vi "Assert To Report Entry.vi"(8 "error in (no error)":errorcluster, 10 "Assert Event Data":T1={"name"="", "passed"=FALSE, "call-chain"=[], "test-error"={"status"=FALSE, "code"=0, "source"=""}, "timestamp"=timestamp(0 s since 1904-01-01), "assert-id"="", "test-id"="", "time"=-1.0, "message"="", "properties"=variant, "measurements"=variant, "user-defined"=variant}) -> (0 "error out":errorcluster, 2 "String":string)   [LabVIEW 2020, in "Caraya.lvlib" / "Test Report.Event.lvclass"]
uses:
  Test Report.Event.lvclass
  Test Report.Event.lvclass/Test Report.Event.ctl
  Test Report/Test Report.lvclass
  Test Result/Assert Event Data (Extended).ctl
  Test Result/Test Result.lvclass
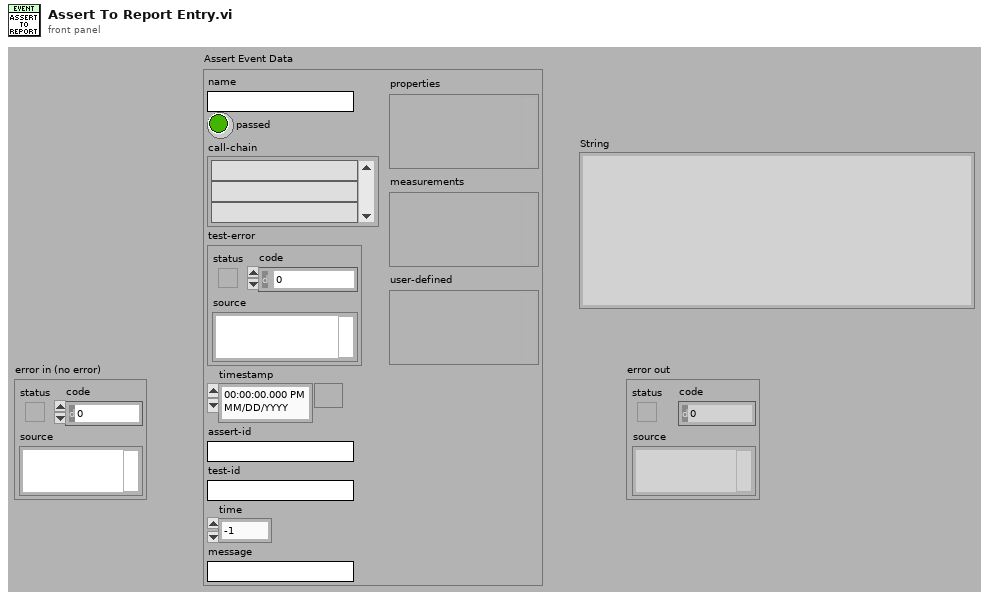
[diagram p1: front panel]
types:
  T1 = typedef "Caraya.lvlib/Test Result.lvclass/Assert Event Data (Extended).ctl" = cluster{"name":string, "passed":bool, "call-chain":string[], "test-error":errorcluster, "timestamp":timestamp, "assert-id":string, "test-id":string, "time":dbl, "message":string, "properties":variant, "measurements":variant, "user-defined":variant}
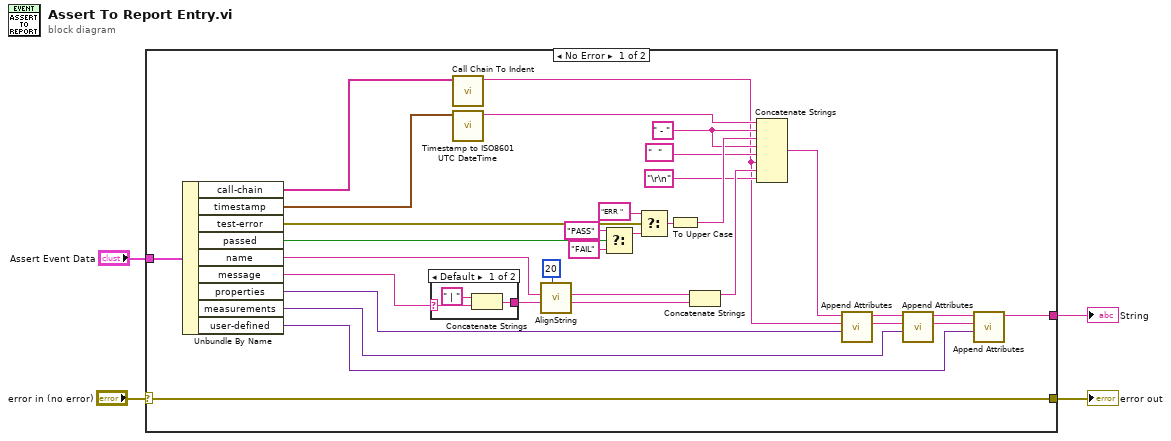
[diagram p0: block diagram]
diagram:
  n1 = case shown="No Error" "error in (no error)" {
    selector: "error in (no error)" -> [w29 w40]
    tunnel: [w29 w40] -> w3
    tunnel: "Assert Event Data" -> [w36 _]
    tunnel: [w7 _] -> w1
    frame No Error {
      w17 = " - " ("string")
      n2 = Unbundle By Name(w36) -> ("call-chain"=w28:string[], "timestamp"=w25:timestamp, "test-error"=w27:errorcluster, "passed"=w26:bool, "name"=w24:string, "message"=w22:string, "properties"=w30:variant, "measurements"=w9:variant, "user-defined"=w5:variant)
      n3 = case shown="Default" w22 {
        selector: w22 -> [w37 _]
        tunnel: [w38 _] -> w21
        frame Default {
          n4 = Concatenate Strings(" | " ("format string"), w37) -> (w38:string)
        }
        frame "" {
        }
      }
      n5 = call "Call Chain To Indent.vi"("Call Chain"=w28) -> ("Indent"=w12:string)  [unwired: 10 in]
      n6 = call <vilib>:"Timestamp to ISO8601 UTC DateTime.vi"("Timestamp (now)"=w25) -> ("ISO8601 UTC DateTime"=w19:string)  [unwired: 10 in]
      n7 = call "AlignString.vi"("min length"=20, "Input"=w24) -> ("Output"=w20:string)  [unwired: 9 in]
      n8 = Select(t="PASS" ("format string"), s=w26, f="FAIL" ("format string")) -> (s? t:f=w32:string)
      n9 = Select(t="ERR " ("format string"), s=w27, f=w32) -> (s? t:f=w33:string)
      n10 = To Upper Case(1:w33) -> (0:w18:string)
      n11 = Concatenate Strings(w20, w21) -> (w15:string)
      n12 = Concatenate Strings(w19, w17, w18, w17, "  " ("string"), w12, w15, "\r\n" ("format string")) -> (w13:string)
      n13 = call "Append Attributes.vi"("attributes"=w30, "Indent"=w12, "String in"=w13) -> ("Indent dup"=w10:string, "String out"=w11:string)  [unwired: 7 in]
      n14 = call "Append Attributes.vi"("attributes"=w9, "Indent"=w10, "String in"=w11) -> ("Indent dup"=w6:string, "String out"=w8:string)  [unwired: 7 in]
      n15 = call "Append Attributes.vi"("attributes"=w5, "Indent"=w6, "String in"=w8) -> ("String out"=w7:string)  [unwired: 7 in, 1 out]
    }
    frame Error {
    }
  }
  "error out" <- w3
  "String" <- w1
